vi "Get Desired Size.vi"(8 "error in (no error)":errorcluster, 11 "BP Item in":refnum<class "BP Item.lvclass">) -> (0 "error out":errorcluster, 2 "Desired Size":T1, 3 "BP Item out":refnum<class "BP Item.lvclass">)   [LabVIEW 2020, in "BP Item.lvclass"]
uses:
  BP Item.lvclass
  lv-oopanel/OOPanel/ArrayPanel/Desired Size.ctl
  lv-oopanel/OOPanel/ArrayPanel/ArrayPanel.lvclass
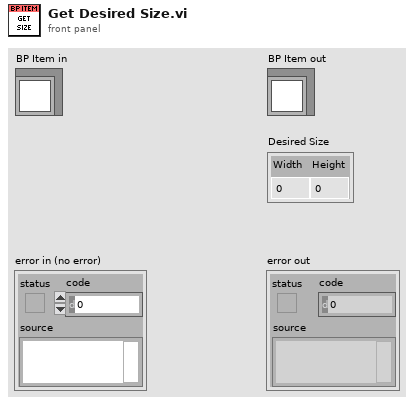
[diagram p1: front panel]
types:
  T1 = typedef "OOPanel.lvlib/ArrayPanel.lvclass/Desired Size.ctl" = cluster{"Width":u32, "Height":u32}
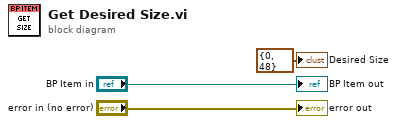
[diagram p0: block diagram]
diagram:
  "error out" <- "error in (no error)"
  "BP Item out" <- "BP Item in"
  "Desired Size" <- T1 {"Width"=0, "Height"=48} ("Desired Size")
